vi "DisplayData.vi"() -> ()   [LabVIEW 2014]
panel:
  out "MX, MY":cluster{dbl[], sgl[]}[](graph)
  out "SA, SB":cluster{dbl[], sgl[]}[](graph)
  out "AY, BY":cluster{dbl[], sgl[]}[](graph)
  out "AX, BX":cluster{dbl[], sgl[]}[](graph)
  in  "file path (use dialog)":path
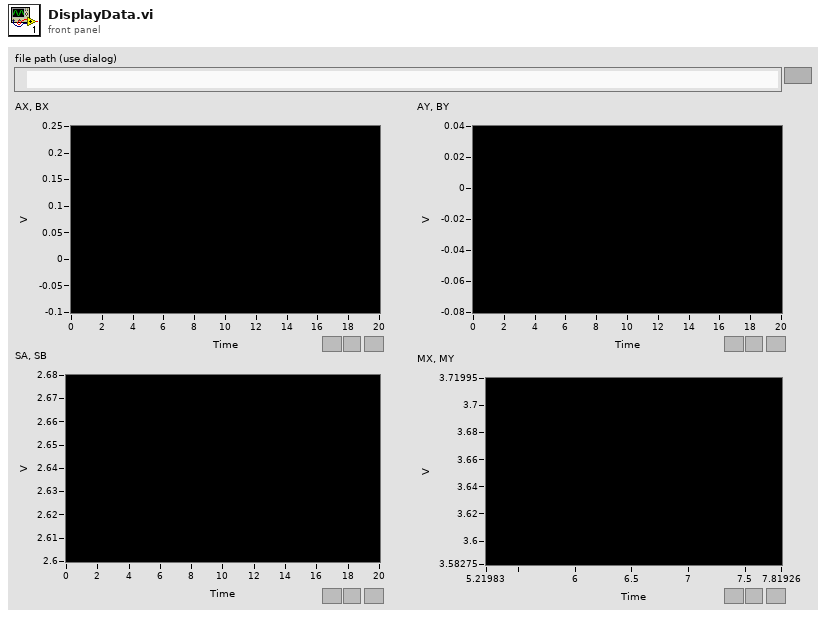
[diagram p1: front panel]
types:
  T1 = enum16{"big-endian, network order", "native, host order", "little-endian"}
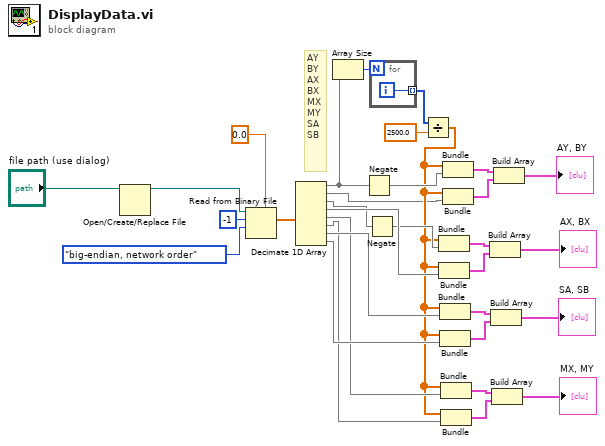
[diagram p0: block diagram]
diagram:
  # "AY\nBY\nAX\nBX\nMX\nMY\nSA\nSB"
  n1 = Open/Create/Replace File(file path (use dialog)="file path (use dialog)") -> (refnum out=w31:refnum<file>)  [unwired: 5 in, 2 out]
  n2 = Read from Binary File(5:sgl 0.0, 9:T1."big-endian, network order" ("byte order (0:big-endian, network order)"), 10:-1 ("count (1)"), 11:w31) -> (2:w27:sgl[])  [unwired: 2 in, 3 out]
  n3 = Decimate 1D Array(w27) -> (w23:sgl[], w4:sgl[], w3:sgl[], w19:sgl[], w9:sgl[], w8:sgl[], w13:sgl[], w14:sgl[])
  n4 = Array Size(array=w23) -> (size(s)=w24:i32)
  n5 = Negate(x=w23) -> (-x=w20:sgl[])
  n6 = Negate(x=w3) -> (-x=w18:sgl[])
  n7 = for {
    N: w24 -> [_]
    tunnel: [w33] -> w7 mode=indexing
    i -> [w33]
  }
  n8 = Divide(x=w7, y=2500.0) -> (x/y=w6:dbl[])
  n9 = Bundle(w6, w18) -> (w21:cluster{dbl[], sgl[]})  [unwired: 1 in]
  n10 = Bundle(w6, w19) -> (w22:cluster{dbl[], sgl[]})  [unwired: 1 in]
  n11 = Bundle(w6, w13) -> (w16:cluster{dbl[], sgl[]})  [unwired: 1 in]
  n12 = Bundle(w6, w14) -> (w15:cluster{dbl[], sgl[]})  [unwired: 1 in]
  n13 = Bundle(w6, w9) -> (w11:cluster{dbl[], sgl[]})  [unwired: 1 in]
  n14 = Bundle(w6, w8) -> (w12:cluster{dbl[], sgl[]})  [unwired: 1 in]
  n15 = Bundle(w6, w20) -> (w26:cluster{dbl[], sgl[]})  [unwired: 1 in]
  n16 = Bundle(w6, w4) -> (w25:cluster{dbl[], sgl[]})  [unwired: 1 in]
  n17 = Build Array(w21, w22) -> (→"AX, BX":cluster{dbl[], sgl[]}[])
  n18 = Build Array(w16, w15) -> (→"SA, SB":cluster{dbl[], sgl[]}[])
  n19 = Build Array(w11, w12) -> (→"MX, MY":cluster{dbl[], sgl[]}[])
  n20 = Build Array(w26, w25) -> (→"AY, BY":cluster{dbl[], sgl[]}[])
